vi "WPI_DigitalOutputConfigurePWMRate.vi"(8 "error in (no error)":errorcluster, 10 "PWM Rate (Hz)":sgl=1000.0) -> (0 "error out":errorcluster, 2 "Actual PWM Rate (Hz)":dbl)   [LabVIEW 2017]
doc: "Specifies the frequency of the PWM signals output by the PWM generator.\n\nThe valid range is from 0.12 Hz to 62.5 kHz. The frequency resolution is logarithmic.\n\nThis software is licensed. Open the labview\\readme\\WPI Robotics Library Open Source License.txt file for more information."
uses:
  <vilib>/Rock Robotics/SystemInterfaces/System/FPGA_SystemGet.vi
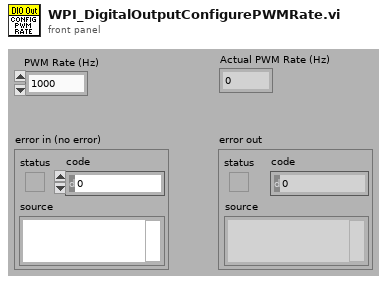
[diagram p1: front panel]
types:
  T1 = typedef "FPGA_DIODevRef.ctl" = cluster{"DevStatus":errorcluster}
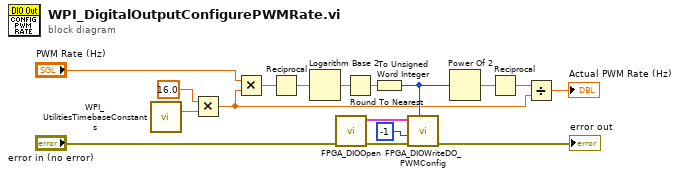
[diagram p0: block diagram]
diagram:
  n1 = call <vilib>:"WPI_UtilitiesTimebaseConstants.vi"() -> ("1 MHz PWM clock"=w14:dbl)  [unwired: 13 in, 2 out]
  n2 = Multiply(x=16.0, y=w14) -> (x*y=w2:dbl)
  n3 = Multiply(x="PWM Rate (Hz)", y=w2) -> (x*y=w15:dbl)
  n4 = Reciprocal(x=w15) -> (1/x=w13:dbl)
  n5 = Logarithm Base 2(1:w13) -> (0:w12:dbl)
  n6 = call <vilib>:"FPGA_DIOOpen.vi"("error in (no error)"="error in (no error)") -> ("error out"=w8:errorcluster, "DIODeviceRef"=w10:T1)  [unwired: 1 in, 8 out]
  n7 = Round To Nearest(number=w12) -> (nearest integer value=w11:dbl)
  n8 = To Unsigned Word Integer(number=w11) -> (unsigned 16bit integer=w7:u16)
  n9 = call <vilib>:"FPGA_DIOWriteDO_PWMConfig.vi"("DO_PWMPeriodPower"=w7, "error in (no error)"=w8, "DO_PWM Index"=i8 -1, "DIODeviceRef"=w10) -> ("error out"=→"error out":errorcluster)  [unwired: 1 in, 6 out]
  n10 = Power Of 2(x=w7) -> (2^x=w6:dbl)
  n11 = Reciprocal(x=w6) -> (1/x=w5:dbl)
  n12 = Divide(x=w5, y=w2) -> (x/y=→"Actual PWM Rate (Hz)":dbl)
